vi "Capture@PatternMatchOne__Parameter.vi"(1 "ParamterIn":string) -> (0 "ParamterOut":string)   [LabVIEW 2019]
uses:
  MainFrame/Global.vi
panel:
  out "Image":T1(plugin-control)
  in  "Picture":string(combo)
  in  "AngleEnd":string(combo)
  in  "AngleStart":string(combo)
  in  "Score":string(combo)
  in  "Point":string(combo)
  in  "CamName":string(combo)
  in  "Confirm":bool
  # "Capture@PatternMatch/GeoMatch $Capture,$Picture,$Score,$Point(,$Angle=XX~XX)"
  # "Angle="
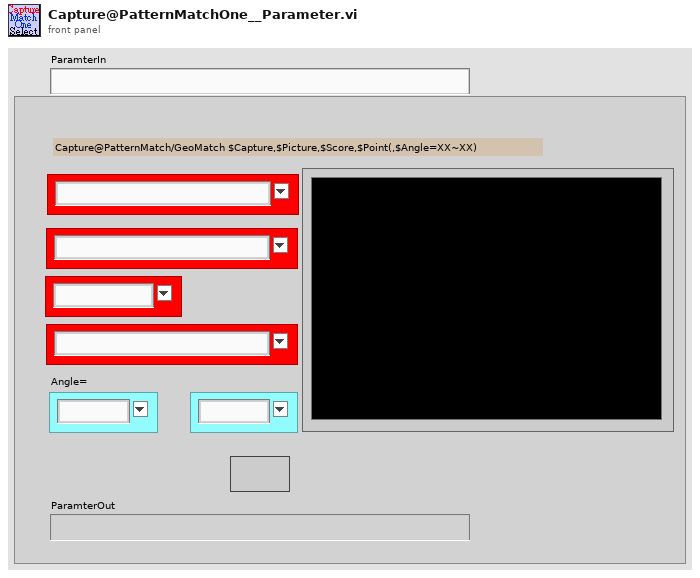
[diagram p1: front panel]
types:
  T1 = typedef "IMAQ Image.ctl" = refnum<image>
  T2 = enum16{"Get", "UpdatePointS", "Init", "UpdateIndex", "GetCurrent&Index+1", "GetWithIndex", "ChkLast", "GetCurrent"}
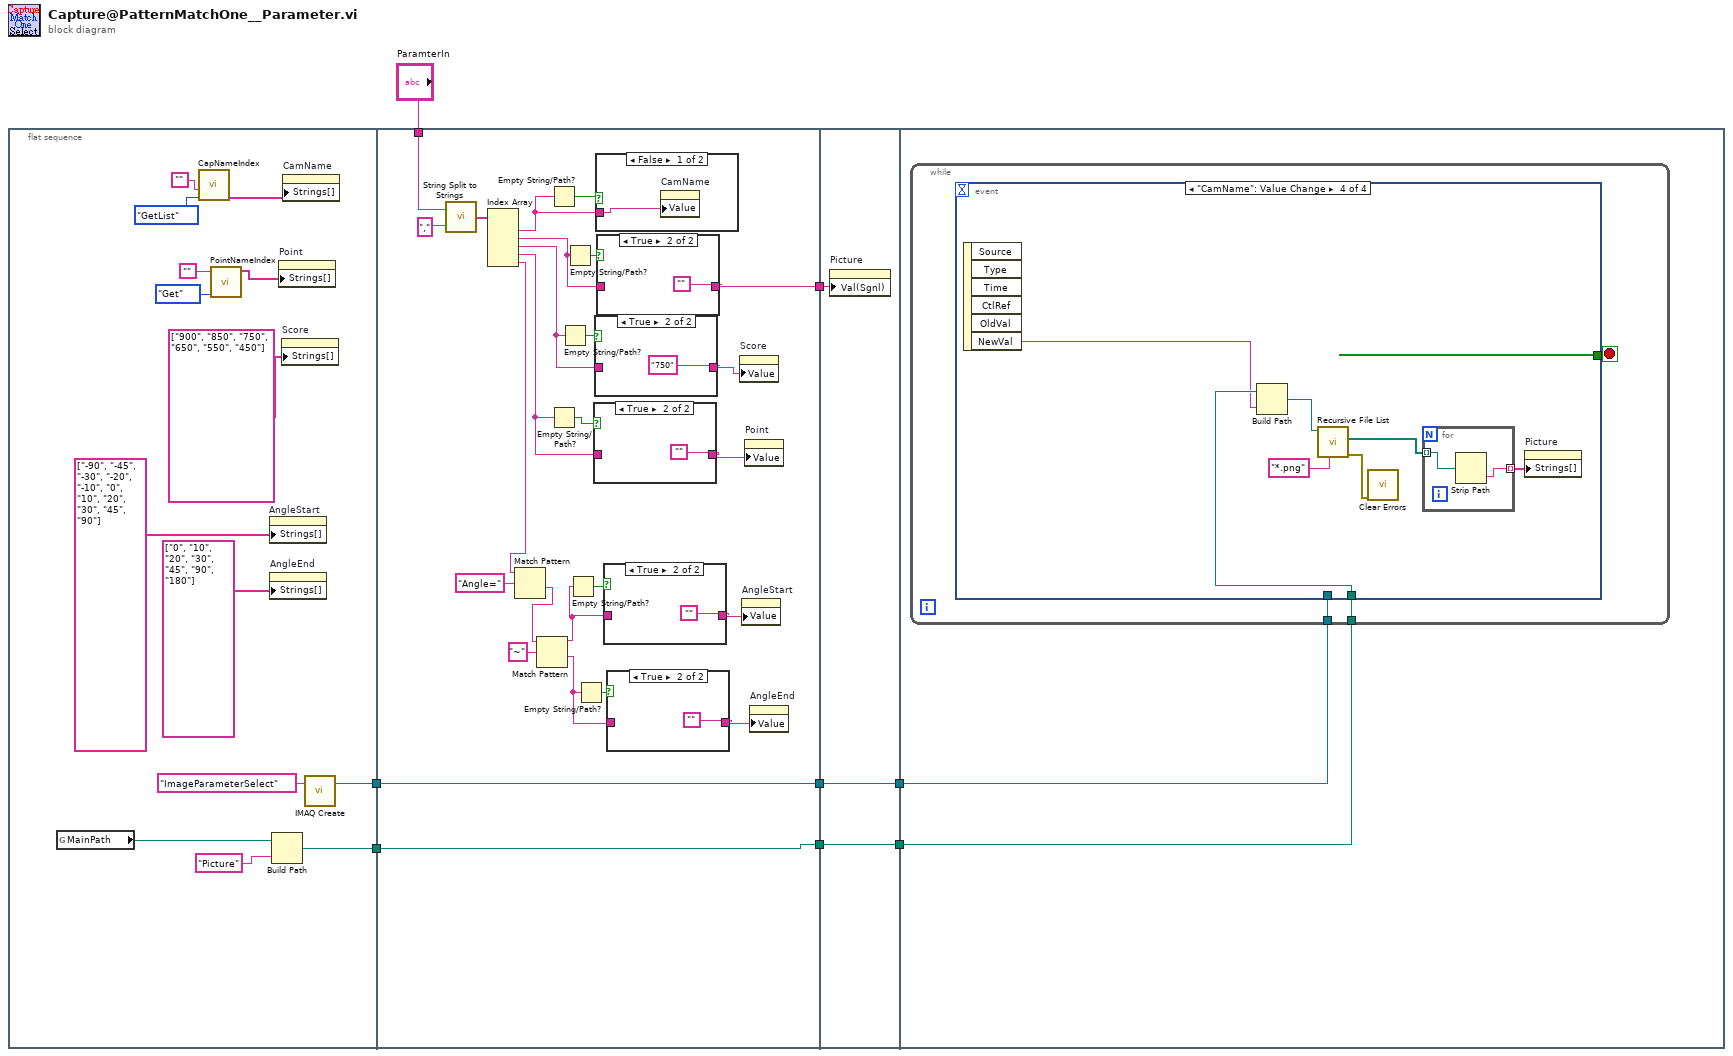
[diagram p0: block diagram]
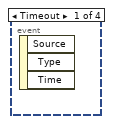
[diagram p8: hidden frame]
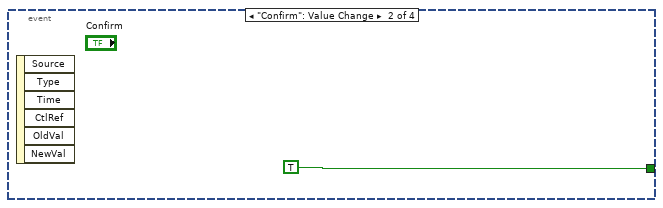
[diagram p9: hidden frame]
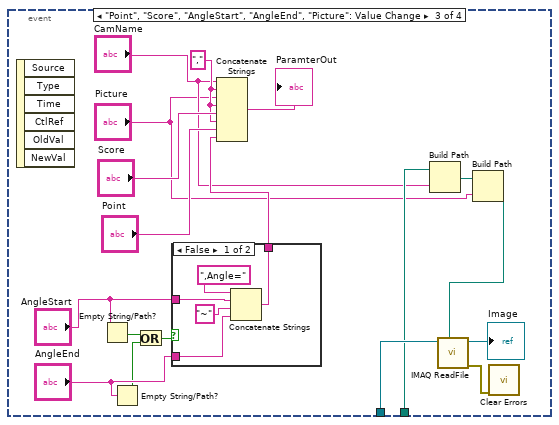
[diagram p10: hidden frame]
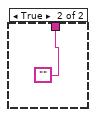
[diagram p11: hidden frame]
diagram:
  n1 = flat-sequence {
    tunnel: [w13] -> w7
    tunnel: [w11] -> w2
    tunnel: "ParamterIn" -> [w46]
    tunnel: w7 -> [w27]
    tunnel: [w27] -> w6
    tunnel: [w25] -> w3
    tunnel: w2 -> [w25]
    tunnel: [w23] -> w1
    tunnel: w6 -> [w62]
    tunnel: [w62] -> w5
    tunnel: [w61] -> w4
    tunnel: w3 -> [w61]
    tunnel: w1 -> [w60]
    tunnel: w5 -> [w64]
    tunnel: w4 -> [w63]
    frame #0 {
      n2 = global read "Global.vi" "MainPath"() -> (w9:path)
      n3 = call "CapNameIndex.vi"("OP"=enum16{"AddCam", "GetIndex", "Init", "GetList"}."GetList", "CamName"="") -> ("DeviceList"=w21:string[])  [unwired: 2 in, 3 out]
      n4 = call "PointNameIndex.vi"("OP"=T2."Get", "PointName"="") -> ("PointNameList"=w17:string[])  [unwired: 4 in, 5 out]
      n5 = property on="AngleStart" class="CmbBox"("Strings[]"=string[] ["-90", "-45", "-30", "-20", "-10", "0", "10", "20", "30", "45", "90"] ("Strings []")) -> ()  [unwired: 2 in, 2 out]
      n6 = property on="AngleEnd" class="CmbBox"("Strings[]"=string[] ["0", "10", "20", "30", "45", "90", "180"] ("Strings []")) -> ()  [unwired: 2 in, 2 out]
      n7 = Build Path(base path=w9, name or relative path="Picture") -> (appended path=w11:path)
      n8 = property on="Point" class="CmbBox"("Strings[]"=w17) -> ()  [unwired: 2 in, 2 out]
      n9 = property on="Score" class="CmbBox"("Strings[]"=string[] ["900", "850", "750", "650", "550", "450"] ("Strings []")) -> ()  [unwired: 2 in, 2 out]
      n10 = property on="CamName" class="CmbBox"("Strings[]"=w21) -> ()  [unwired: 2 in, 2 out]
      n11 = call "IMAQ Create"("Image Name"="ImageParameterSelect") -> ("New Image"=w13:T1)  [unwired: 4 in, 1 out]
    }
    frame #1 {
      n12 = call "String Split to Strings.vi"("search string/char (-)"=",", "String"=w46) -> ("Array"=w48:string[])
      n13 = Index Array(array=w48) -> (element #1=w26:string, element #2=w38:string, element #3=w41:string, element #4=w43:string, element #5=w37:string)  [unwired: 5 in]
      n14 = Match Pattern(string=w37, regular expression="Angle=") -> (after substring=w35:string)  [unwired: 1 in, 3 out]
      n15 = Match Pattern(string=w35, regular expression="~") -> (before substring=w32:string, after substring=w30:string)  [unwired: 1 in, 2 out]
      n16 = Empty String/Path?(string/path=w26) -> (empty?=w45:bool)
      n17 = Empty String/Path?(string/path=w43) -> (empty?=w44:bool)
      n18 = Empty String/Path?(string/path=w41) -> (empty?=w42:bool)
      n19 = Empty String/Path?(string/path=w38) -> (empty?=w39:bool)
      n20 = Empty String/Path?(string/path=w32) -> (empty?=w33:bool)
      n21 = Empty String/Path?(string/path=w30) -> (empty?=w31:bool)
      n22 = case shown="True" w44 {
        tunnel: [w57 ""] -> w24
        tunnel: w43 -> [w57 _]
        frame False {
        }
        frame True {
        }
      }
      n23 = case shown="True" w42 {
        tunnel: [w55 "750"] -> w40
        tunnel: w41 -> [w55 _]
        frame False {
        }
        frame True {
        }
      }
      n24 = case shown="False" w45 {
        tunnel: w26 -> [w59 _]
        frame False {
          n25 = property on="CamName" class="CmbBox"("Value"=w59) -> ()  [unwired: 2 in, 2 out]
        }
        frame True {
        }
      }
      n26 = case shown="True" w39 {
        tunnel: [w53 ""] -> w23
        tunnel: w38 -> [w53 _]
        frame False {
        }
        frame True {
        }
      }
      n27 = case shown="True" w33 {
        tunnel: [w51 ""] -> w29
        tunnel: w32 -> [w51 _]
        frame False {
        }
        frame True {
        }
      }
      n28 = case shown="True" w31 {
        tunnel: [w49 ""] -> w28
        tunnel: w30 -> [w49 _]
        frame False {
        }
        frame True {
        }
      }
      n29 = property on="Score" class="CmbBox"("Value"=w40) -> ()  [unwired: 2 in, 2 out]
      n30 = property on="AngleStart" class="CmbBox"("Value"=w29) -> ()  [unwired: 2 in, 2 out]
      n31 = property on="Point" class="CmbBox"("Value"=w24) -> ()  [unwired: 2 in, 2 out]
      n32 = property on="AngleEnd" class="CmbBox"("Value"=w28) -> ()  [unwired: 2 in, 2 out]
    }
    frame #2 {
      n33 = property on="Picture" class="CmbBox"("Val(Sgnl)"=w60) -> ()  [unwired: 2 in, 2 out]
    }
    frame #3 {
      n34 = while {
        tunnel: w64 -> [w66]
        tunnel: w63 -> [w65]
        stop <- w67 stop-if-true
        n35 = event shown="[3] \"CamName\": Value Change" {
          selector: _ -> [_ _ _ _]
          dyn-events: _ -> [_ _ _ _]
          timeout: _ -> [_ _ _ _]
          tunnel: [_ TRUE _ _] -> w67
          tunnel: w66 -> [_ _ w76 _]
          tunnel: w65 -> [_ _ w75 w96]
          event Timeout {
            n36 = event-data() -> ()  [unwired: 1 in, 3 out]
          }
          event "Confirm": Value Change {
            n37 = event-data() -> ()  [unwired: 1 in, 6 out]
          }
          event "Point", "Score", "AngleStart", "AngleEnd", "Picture": Value Change {
            w83 = "," ("string")
            n38 = event-data() -> ()  [unwired: 1 in, 6 out]
            n39 = Empty String/Path?(string/path="AngleStart") -> (empty?=w78:bool)
            n40 = Empty String/Path?(string/path="AngleEnd") -> (empty?=w77:bool)
            n41 = Or(x=w78, y=w77) -> (x .or. y?=w79:bool)
            n42 = case shown="False" w79 {
              tunnel: [w89 ""] -> w82
              tunnel: "AngleStart" -> [w88 _]
              tunnel: "AngleEnd" -> [w87 _]
              frame False {
                n43 = Concatenate Strings(",Angle=" ("string"), w88, "~", w87) -> (w89:string)
              }
              frame True {
              }
            }
            n44 = Concatenate Strings("CamName", w83, "Picture", w83, "Score", w83, "Point", w82) -> (→"ParamterOut":string)
            n45 = Build Path(base path=w75, name or relative path="CamName") -> (appended path=w73:path)
            n46 = Build Path(base path=w73, name or relative path="Picture") -> (appended path=w71:path)
            n47 = call "IMAQ ReadFile"("File Path"=w71, "Image"=w76) -> ("error out"=w70:errorcluster, "Image Out"=→"Image":T1)  [unwired: 5 in, 3 out]
            n48 = call <vilib>:"Clear Errors.vi"("error in (no error)"=w70) -> ()  [unwired: 5 in, 2 out]
          }
          event "CamName": Value Change {
            n49 = event-data() -> ("NewVal"=w95:string)  [unwired: 1 in, 5 out]
            n50 = Build Path(base path=w96, name or relative path=w95) -> (appended path=w94:path)
            n51 = call <vilib>:"Recursive File List.vi"("pattern"="*.png", "Folder Path"=w94) -> ("error out"=w93:errorcluster, "All Files in Dir"=w98:path[])  [unwired: 5 in, 3 out]
            n52 = call <vilib>:"Clear Errors.vi"("error in (no error)"=w93) -> ()  [unwired: 5 in, 2 out]
            n53 = for {
              tunnel: w98 -> [w101] mode=indexing
              tunnel: [w100] -> w99 mode=indexing
              n54 = Strip Path(path=w101) -> (name=w100:string)  [unwired: 1 out]
            }
            n55 = property on="Picture" class="CmbBox"("Strings[]"=w99) -> ()  [unwired: 2 in, 2 out]
          }
        }
      }
    }
  }
